vi "convert sdi to xml encoding (ni).vi"(11 "SDI":i32) -> (3 "xml sdi format":i32)   [LabVIEW 2020]
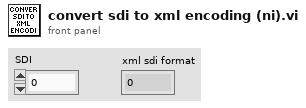
[diagram p1: front panel]
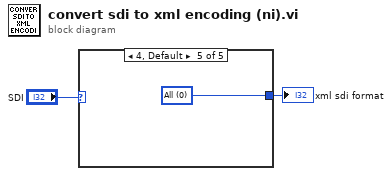
[diagram p0: block diagram]
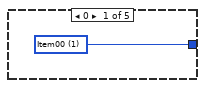
[diagram p2: hidden frame]
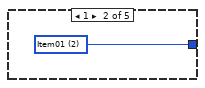
[diagram p3: hidden frame]
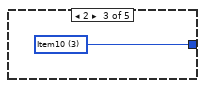
[diagram p4: hidden frame]
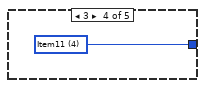
[diagram p5: hidden frame]
diagram:
  n1 = case shown="4, Default" "SDI" {
    tunnel: [w3 w4 w5 w6 w7] -> w1
    frame 0 {
      w3 = 1 items=["All", "Item00", "Item01", "Item10", "Item11"] ("sdi")
    }
    frame 1 {
      w4 = 2 items=["All", "Item00", "Item01", "Item10", "Item11"] ("sdi")
    }
    frame 2 {
      w5 = 3 items=["All", "Item00", "Item01", "Item10", "Item11"] ("sdi")
    }
    frame 3 {
      w6 = 4 items=["All", "Item00", "Item01", "Item10", "Item11"] ("sdi")
    }
    frame 4, Default {
      w7 = 0 items=["All", "Item00", "Item01", "Item10", "Item11"] ("sdi")
    }
  }
  "xml sdi format" <- w1
